vi "FaradayCup_Lock_Unlock.vi"(8 "entrée d'erreur (pas d'erreur)":errorcluster, 10 "Control-Client old entrée":refnum<class "Control-Client.lvclass">, 11 "Control-Client new entrée":refnum<class "Control-Client.lvclass">) -> (0 "sortie d'erreur":errorcluster caption="entrée d'erreur (pas d'erreur)")   [LabVIEW 2015, in "Control-Client.lvclass"]
uses:
  Control-Client.lvclass
  Control-Client.lvclass/Control-Client.ctl
  dependecies/XControls/CellsDL/ControlDL.xctl
  controls/Gauge_pump/Gauge_pump.xctl
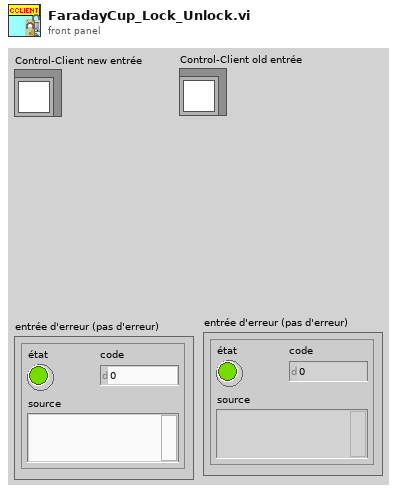
[diagram p1: front panel]
types:
  T1 = enum8{"Enabled", "Disabled", "Disabled and Grayed Out"}
  T2 = typedef "Control-Client.lvclass/Controls-with-permissions_CLIENT.ctl" = cluster{"Server ON/OFF":refnum<vi>, "Detector connect":refnum<vi>, "DL connect":refnum<vi>, "DAQmx connect":refnum<vi>, "All connect":refnum<vi>, "Start measurement":refnum<vi>, "Move Crystal":refnum<vi>, "Relay key heater":refnum<vi>, "Laser Shutter":refnum<vi>, "Accelerator Shutter":refnum<vi>, "Power":refnum<vi>, "Unlock":refnum<vi>, "RT":refnum<vi>, "Faraday Cup":refnum<vi>, "Osc connect":refnum<vi>, "ELYSE pulses":refnum<vi>, "Cells":refnum<vi>, "ControlDL":refnum<vi>, "Pump":refnum<vi>, "# par point":refnum<vi>, "Alarm":refnum<vi>, "oscilloscopeRead":refnum<vi>, "WCM_state":refnum<vi>}
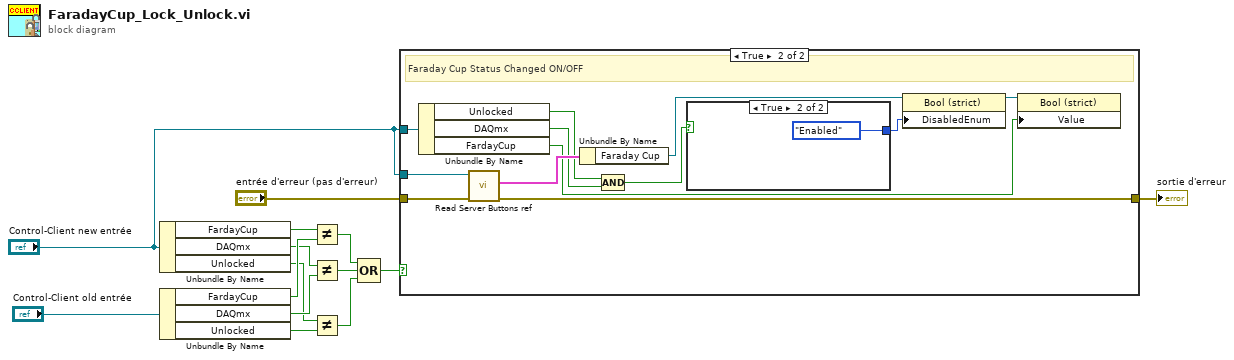
[diagram p0: block diagram]
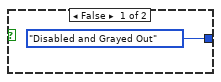
[diagram p3: hidden frame]
diagram:
  n1 = Unbundle By Name("Control-Client new entrée") -> ("FardayCup"=w9:bool, "DAQmx"=w8:bool, "Unlocked"=w2:bool)
  n2 = Unbundle By Name("Control-Client old entrée") -> ("FardayCup"=w10:bool, "DAQmx"=w7:bool, "Unlocked"=w1:bool)
  n3 = Not Equal?(x=w9, y=w10) -> (x != y?=w6:bool)
  n4 = Not Equal?(x=w8, y=w7) -> (x != y?=w5:bool)
  n5 = Not Equal?(x=w2, y=w1) -> (x != y?=w3:bool)
  n6 = Compound Arithmetic op=OR ("Opérateur arithmétique")(w6, w5, w3) -> (w4:bool)
  n7 = case shown="True" w4 {
    tunnel: "Control-Client new entrée" -> [_ w27]
    tunnel: [w15 w23] -> w13
    tunnel: "entrée d'erreur (pas d'erreur)" -> [w15 w22]
    tunnel: "Control-Client new entrée" -> [_ w19]
    frame False {
    }
    frame True {
      # "Faraday Cup Status Changed ON/OFF"
      n8 = Unbundle By Name(w19) -> ("Unlocked"=w17:bool, "DAQmx"=w18:bool, "FardayCup"=w16:bool)
      n9 = call "Read Server Buttons ref.vi"("error in (no error)"=w22, "Control-Client in"=w27) -> ("error out"=w23:errorcluster, "Server Buttons ref"=w25:T2)  [unwired: 7 in, 1 out]
      n10 = Unbundle By Name(w25) -> ("Faraday Cup"=w26:refnum<vi>)
      n11 = Compound Arithmetic op=AND(w17, w18) -> (w21:bool)
      n12 = case shown="True" w21 {
        tunnel: [T1."Disabled and Grayed Out" ("Désactivé") T1."Enabled" ("Désactivé")] -> w24
        frame False {
        }
        frame True {
        }
      }
      n13 = property class="Bool (strict)"(reference=w26, "DisabledEnum"=w24) -> (reference out=w20:refnum<vi>)  [unwired: 1 in, 1 out]
      n14 = property class="Bool (strict)"(reference=w20, "Value"=w16) -> ()  [unwired: 1 in, 2 out]
    }
  }
  "sortie d'erreur" <- w13
